vi "Address Claim.vi"(8 "error in (no error)":errorcluster, 11 "J1939 Main Configuration":T1={"Parameters"={"J1939 XNET Settings"={"XNET Database"="", "XNET Cluster"="", "CAN Port"="", "Baud rate [Bd]"=0, "Termination"=0, "Incoming Rate"=0, "Outcoming Rate"=1, "Write Decimation"=1}, "Incoming Single Point Configuraiton"={"Incoming Single Point Frame"={"ID"=[], "Conversion"=[], "Channel Array Positions"=[], "Frame Length"=[]}, "Channel Pairs"={"Chan Refs"=[], "Previous Chan Values"=[]}, "Read FIFO"=refnum}, "Outgoing Cyclic Configuraiton"={"Outgoing Cyclic Frame"={"ID"=[], "Conversion"=[], "Channel Array Positions"=[], "Frame Length"=[], "Transmit Propreties"=[]}, "Channel Pairs"={"Block Data Refs"=[], "Previous Chan Values"=[]}, "Write FIFO"=refnum}, "J1939 Monitor Settings"={"J1939 Network Address"=0, "Name"=0}, "Simulated Addresses"=[], "Simulated Addresses LUT"=variant, "Name"=""}, "Name"="", "J1939 Cluster"={"Processed Incoming"=refnum, "Current Device Address"=0, "Processed Outgoing"=refnum, "Process Outgoing"=refnum, "Name"=0}, "References"={"BAM Buffer"=refnum, "CM Buffer"=refnum, "CM Gen"=refnum, "BAM Gen"=refnum, "Address Claims"=refnum, "RQST"=refnum}, "Frame In"="", "Frame Out"="", "Incoming Timeout"=0, "Outgoing Timeout"=0, "Listener ID"=refnum, "Process"=refnum, "Data Ref"=refnum, "Scale Ref"=refnum, "Incoming Direct Access"={"Offset"=0, "Length"=0}, "Outgoing Direct Access"={"Offset"=0, "Length"=0}, "TCP Mngr Ref"=refnum, "Name and Address"="", "Simulated Addresses"=[], "Simulated Addresses LUT"=variant} {"Simulated Addresses"."Simulated Addresses"."J1939 XNET Settings"."Name" format="%.0x"; "Simulated Addresses"."Simulated Addresses"."DM1 Data"."Data Reference" format="%.0x"; "Simulated Addresses"."Simulated Addresses"."DM1 Enable?"."Data Reference" format="%.0x"; "Simulated Addresses"."Simulated Addresses"."DM2 Data"."Data Reference" format="%.0x"; "Simulated Addresses"."Simulated Addresses"."DM2 Enable?"."Data Reference" format="%.0x"; "Parameters"."Simulated Addresses"."Simulated Addresses"."J1939 XNET Settings"."Name" format="%.0x"; "Parameters"."J1939 Monitor Settings"."Name" format="%.0x"; "Parameters"."Outgoing Cyclic Configuraiton"."Channel Pairs"."Block Data Refs"."Data Reference" format="%.0x"; "Parameters"."Outgoing Cyclic Configuraiton"."Outgoing Cyclic Frame"."Transmit Propreties"."Transmit Time" format="%#_p"; "Parameters"."J1939 XNET Settings"."Termination" items=["Off", "On"]; "Parameters"."Incoming Single Point Configuraiton"."Channel Pairs"."Chan Refs" format="%.0x"}) -> (0 "error out":errorcluster, 3 "J1939 Main Configuration Out":T1={"Parameters"={"J1939 XNET Settings"={"XNET Database"="", "XNET Cluster"="", "CAN Port"="", "Baud rate [Bd]"=0, "Termination"=0, "Incoming Rate"=0, "Outcoming Rate"=1, "Write Decimation"=1}, "Incoming Single Point Configuraiton"={"Incoming Single Point Frame"={"ID"=[], "Conversion"=[], "Channel Array Positions"=[], "Frame Length"=[]}, "Channel Pairs"={"Chan Refs"=[], "Previous Chan Values"=[]}, "Read FIFO"=refnum}, "Outgoing Cyclic Configuraiton"={"Outgoing Cyclic Frame"={"ID"=[], "Conversion"=[], "Channel Array Positions"=[], "Frame Length"=[], "Transmit Propreties"=[]}, "Channel Pairs"={"Block Data Refs"=[], "Previous Chan Values"=[]}, "Write FIFO"=refnum}, "J1939 Monitor Settings"={"J1939 Network Address"=0, "Name"=0}, "Simulated Addresses"=[], "Simulated Addresses LUT"=variant, "Name"=""}, "Name"="", "J1939 Cluster"={"Processed Incoming"=refnum, "Current Device Address"=0, "Processed Outgoing"=refnum, "Process Outgoing"=refnum, "Name"=0}, "References"={"BAM Buffer"=refnum, "CM Buffer"=refnum, "CM Gen"=refnum, "BAM Gen"=refnum, "Address Claims"=refnum, "RQST"=refnum}, "Frame In"="", "Frame Out"="", "Incoming Timeout"=0, "Outgoing Timeout"=0, "Listener ID"=refnum, "Process"=refnum, "Data Ref"=refnum, "Scale Ref"=refnum, "Incoming Direct Access"={"Offset"=0, "Length"=0}, "Outgoing Direct Access"={"Offset"=0, "Length"=0}, "TCP Mngr Ref"=refnum, "Name and Address"="", "Simulated Addresses"=[], "Simulated Addresses LUT"=variant} {"Simulated Addresses"."Simulated Addresses"."J1939 XNET Settings"."Name" format="%.0x"; "Simulated Addresses"."Simulated Addresses"."DM1 Data"."Data Reference" format="%.0x"; "Simulated Addresses"."Simulated Addresses"."DM1 Enable?"."Data Reference" format="%.0x"; "Simulated Addresses"."Simulated Addresses"."DM2 Data"."Data Reference" format="%.0x"; "Simulated Addresses"."Simulated Addresses"."DM2 Enable?"."Data Reference" format="%.0x"; "Parameters"."Simulated Addresses"."Simulated Addresses"."J1939 XNET Settings"."Name" format="%.0x"; "Parameters"."J1939 Monitor Settings"."Name" format="%.0x"; "Parameters"."Outgoing Cyclic Configuraiton"."Channel Pairs"."Block Data Refs"."Data Reference" format="%.0x"; "Parameters"."Outgoing Cyclic Configuraiton"."Outgoing Cyclic Frame"."Transmit Propreties"."Transmit Time" format="%#_p"; "Parameters"."J1939 XNET Settings"."Termination" items=["Off", "On"]; "Parameters"."Incoming Single Point Configuraiton"."Channel Pairs"."Chan Refs" format="%.0x"})   [LabVIEW 2015, in "J1939 Addon Engine.lvlib"]
uses:
  J1939 Addon Engine.lvlib
  Types/Configuration Cluster.ctl
  <vilib>/NI/NI VeriStand Inline Async API/_VS Inline Async API/Process/Process.lvclass
  Types/Process Parameters.ctl
  Shared/Types/XNET Settings.ctl
  Types/Incoming Single Point Configuration.ctl
  Types/Incoming Single Point Frame Pairs.ctl
  Shared/Types/Incoming Single Point Channel Pairs.ctl
  <vilib>/NI Veristand/Custom Device API/Data Reference.ctl
  Types/Outgoing Cyclic Configuration.ctl
  Types/Outgoing Cyclic Frame Pairs.ctl
  Shared/Types/XNET Frame Event Properties.ctl
  Shared/Types/Outgoing Cyclic Channel Pairs.ctl
  <vilib>/NI Veristand/Custom Device API/Block Data Reference.ctl
  Shared/Types/Monitor Settings.ctl
  Types/Simulated Settings.ctl
  Shared/Types/Compiled Simulated Settings.ctl
  Types/DTC FIFOs.ctl
  Types/Setup Information Cluster.ctl
  <vilib>/xnet/xnet.llb/XNET Frame CAN.ctl
  <vilib>/xnet/xnet.llb/XNET Frame Type CAN.ctl
  Shared/J1939 Utilities/Types/CAN Outgoing Message Cluster.ctl
  Types/TP List References.ctl
  Types/BAM Buffer Connections List_Ref.ctl
  Types/TP Buffer Connection Cluster.ctl
  Types/Connection Mode Generation Connection Ref.ctl
  Types/Connection Mode Generation Connection Cluster.ctl
  Types/BAM Generation Connections List_Ref.ctl
  Types/BAM Generation Connection Cluster.ctl
  Types/Address Table Reference.ctl
  Types/RQST Lookup Table Reference.ctl
  Types/Data Lookup Table Reference.ctl
  Types/Datatable Lookup DVR.ctl
  Types/Conversion Lookup Table Reference.ctl
  Shared/Types/RQST Comm Lookup Table_Ref.ctl
  Shared/STM/Connection Manager/stm_ManagerStateVariables.ctl
  Shared/STM/TCP/stm_TCP Connection Info.ctl
  Shared/STM/_SubVIs/stm_MetaDataElement.ctl
  Shared/STM/Connection Manager/stm_TCPConnectionProperties.ctl
  Types/Address Lookup Table Action.ctl
  Shared/J1939 Utilities/SubVIs/Convert CAN Data (U8) to U32.vi
  Shared/J1939 Utilities/SubVIs/Convert CAN Data (U32) to U8.vi
  Shared/J1939 Utilities/SubVIs/Convert CAN Arb ID to J1939 ID.vi
  Shared/J1939 Utilities/SubVIs/Convert J1939 ID to CAN Arb ID.vi
  <vilib>/xnet/xnet.llb/XNET Write (Frame CAN).vi
  SubVIs/Address Lookup Table.vi
  <vilib>/xnet/xnet.llb/XNET Read.vi
  <vilib>/xnet/xnet.llb/XNET Read (Frame CAN).vi
  Shared/J1939 Utilities/SubVIs/Request Address.vi
  Shared/J1939 Utilities/J1939 Utilities.lvlib
  <vilib>/NI Veristand/Custom Device Tools/Custom Device Utility Library/Custom Device Utility Library.lvlib
  <vilib>/NI VeriStand/Custom Device API/Custom Device API.lvlib
  Shared/J1939 Addon Shared.lvlib
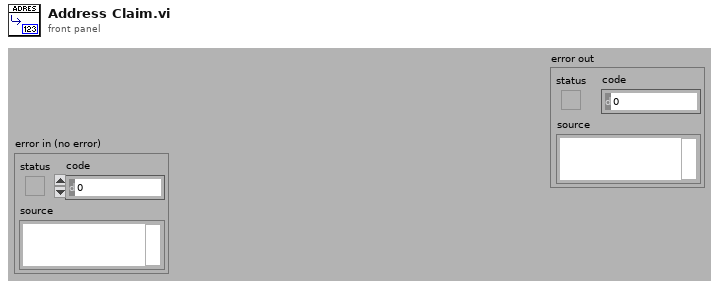
[diagram p1: front panel]
types:
  T1 = typedef "J1939 Addon Engine.lvlib/Configuration Cluster.ctl" = cluster{"Parameters":T2, "Name":string, "J1939 Cluster":T17, "References":T18, "Frame In":refnum<k21>, "Frame Out":refnum<k21>, "Incoming Timeout":u32, "Outgoing Timeout":u32, "Listener ID":refnum<k5>, "Process":refnum<class "Process.lvclass">, "Data Ref":T24, "Scale Ref":T25, "Incoming Direct Access":cluster{"Offset":u32, "Length":u32}, "Outgoing Direct Access":cluster{"Offset":u32, "Length":u32}, "TCP Mngr Ref":T26, "Name and Address":string, "Simulated Addresses":T14[], "Simulated Addresses LUT":variant}
  T2 = typedef "J1939 Addon Engine.lvlib/Process Parameters.ctl" = cluster{"J1939 XNET Settings":T3, "Incoming Single Point Configuraiton":T4, "Outgoing Cyclic Configuraiton":T8, "J1939 Monitor Settings":T13, "Simulated Addresses":T14[], "Simulated Addresses LUT":variant, "Name":string}
  T3 = typedef "J1939 Addon Shared.lvlib/XNET Settings.ctl" = cluster{"XNET Database":refnum<k21>, "XNET Cluster":refnum<k21>, "CAN Port":string, "Baud rate [Bd]":u32, "Termination":u32, "Incoming Rate":u32, "Outcoming Rate":u32, "Write Decimation":u32}
  T4 = typedef "J1939 Addon Engine.lvlib/Incoming Single Point Configuration.ctl" = cluster{"Incoming Single Point Frame":T5, "Channel Pairs":T6, "Read FIFO":refnum<k33>}
  T5 = typedef "J1939 Addon Engine.lvlib/Incoming Single Point Frame Pairs.ctl" = cluster{"ID":u32[], "Conversion":refnum<k21>[], "Channel Array Positions":cluster{"Offset":u32, "Length":u32}[], "Frame Length":u32[]}
  T6 = typedef "J1939 Addon Shared.lvlib/Incoming Single Point Channel Pairs.ctl" = cluster{"Chan Refs":T7[], "Previous Chan Values":dbl[]}
  T7 = typedef "Custom Device API.lvlib/Data Reference.ctl" = i32
  T8 = typedef "J1939 Addon Engine.lvlib/Outgoing Cyclic Configuration.ctl" = cluster{"Outgoing Cyclic Frame":T9, "Channel Pairs":T11, "Write FIFO":refnum<k33>}
  T9 = typedef "J1939 Addon Engine.lvlib/Outgoing Cyclic Frame Pairs.ctl" = cluster{"ID":u32[], "Conversion":refnum<k21>[], "Channel Array Positions":cluster{"Offset":u32, "Length":u32}[], "Frame Length":u32[], "Transmit Propreties":T10[]}
  T10 = typedef "J1939 Addon Shared.lvlib/XNET Frame Event Properties.ctl" = cluster{"Transmit trigger":enum16{"Channel value change"}, "Enable software cyclic trigger":bool, "Transmit Time":dbl}
  T11 = typedef "J1939 Addon Shared.lvlib/Outgoing Cyclic Channel Pairs.ctl" = cluster{"Block Data Refs":T12[], "Previous Chan Values":dbl[]}
  T12 = typedef "Custom Device API.lvlib/Block Data Reference.ctl" = cluster{"Data Reference":T7, "Offset":u64, "Length":u64}
  T13 = typedef "J1939 Addon Shared.lvlib/Monitor Settings.ctl" = cluster{"J1939 Network Address":u8, "Name":u64}
  T14 = typedef "J1939 Addon Engine.lvlib/Simulated Settings.ctl" = cluster{"Simulated Addresses":T15, "FIFOs":T16}
  T15 = typedef "J1939 Addon Shared.lvlib/Compiled Simulated Settings.ctl" = cluster{"J1939 XNET Settings":T13, "DM1 Data":T12[], "DM1 Data":dbl[], "DM1 Enable?":T12[], "DM1 Enable?":dbl[], "DM2 Data":T12[], "DM2 Data":dbl[], "DM2 Enable?":T12[], "DM2 Enable?":dbl[]}
  T16 = typedef "J1939 Addon Engine.lvlib/DTC FIFOs.ctl" = cluster{"DM1 Data":refnum<k33>, "DM1 Enable?":refnum<k33>, "DM2 Data":refnum<k33>, "DM2 Enable?":refnum<k33>, "DM1 Reset?":refnum<k33>, "DM2 Reset?":refnum<k33>}
  T17 = typedef "J1939 Addon Engine.lvlib/Setup Information Cluster.ctl" = cluster{"Processed Incoming":refnum<queue>, "Current Device Address":u8, "Processed Outgoing":refnum<queue>, "Process Outgoing":refnum<queue>, "Name":u64}
  T18 = typedef "J1939 Addon Engine.lvlib/TP List References.ctl" = cluster{"BAM Buffer":T19, "CM Buffer":T19, "CM Gen":T20, "BAM Gen":T21, "Address Claims":T22, "RQST":T23}
  T19 = typedef "J1939 Addon Engine.lvlib/BAM Buffer Connections List_Ref.ctl" = refnum<data-value>
  T20 = typedef "J1939 Addon Engine.lvlib/Connection Mode Generation Connection Ref.ctl" = refnum<data-value>
  T21 = typedef "J1939 Addon Engine.lvlib/BAM Generation Connections List_Ref.ctl" = refnum<data-value>
  T22 = typedef "J1939 Addon Engine.lvlib/Address Table Reference.ctl" = refnum<data-value>
  T23 = typedef "J1939 Addon Engine.lvlib/RQST Lookup Table Reference.ctl" = refnum<data-value>
  T24 = typedef "J1939 Addon Engine.lvlib/Data Lookup Table Reference.ctl" = refnum<data-value>
  T25 = typedef "J1939 Addon Engine.lvlib/Conversion Lookup Table Reference.ctl" = refnum<data-value>
  T26 = typedef "J1939 Addon Shared.lvlib/RQST Comm Lookup Table_Ref.ctl" = refnum<data-value>
  T27 = typedef "J1939 Addon Shared.lvlib/J1939 Utilities.lvlib/CAN Outgoing Message Cluster.ctl" = cluster{"Identifier":u32, "Data":u8[]}
  T28 = typedef "XNET Frame CAN.ctl" = cluster{"timestamp":timestamp, "payload":u8[], "identifier":u32, "type":T29, "extended?":bool, "echo?":bool}
  T29 = typedef "XNET Frame Type CAN.ctl" = u8
  T30 = typedef "J1939 Addon Shared.lvlib/J1939 Utilities.lvlib/Convert CAN Data (U8) Cluster.ctl" = cluster{"Byte 1":u8, "Byte 2":u8, "Byte 3":u8, "Byte 4":u8, "Byte 5":u8, "Byte 6":u8, "Byte 7":u8, "Byte 8":u8}
  T31 = typedef "J1939 Addon Engine.lvlib/Address Lookup Table Action.ctl" = enum16{"Initialize", "Add", "Get", "Remove", "Get All"}
  T32 = typedef "J1939 Addon Shared.lvlib/Address Lookup Table Data.ctl" = cluster{"Name":u8[], "Address":u8}
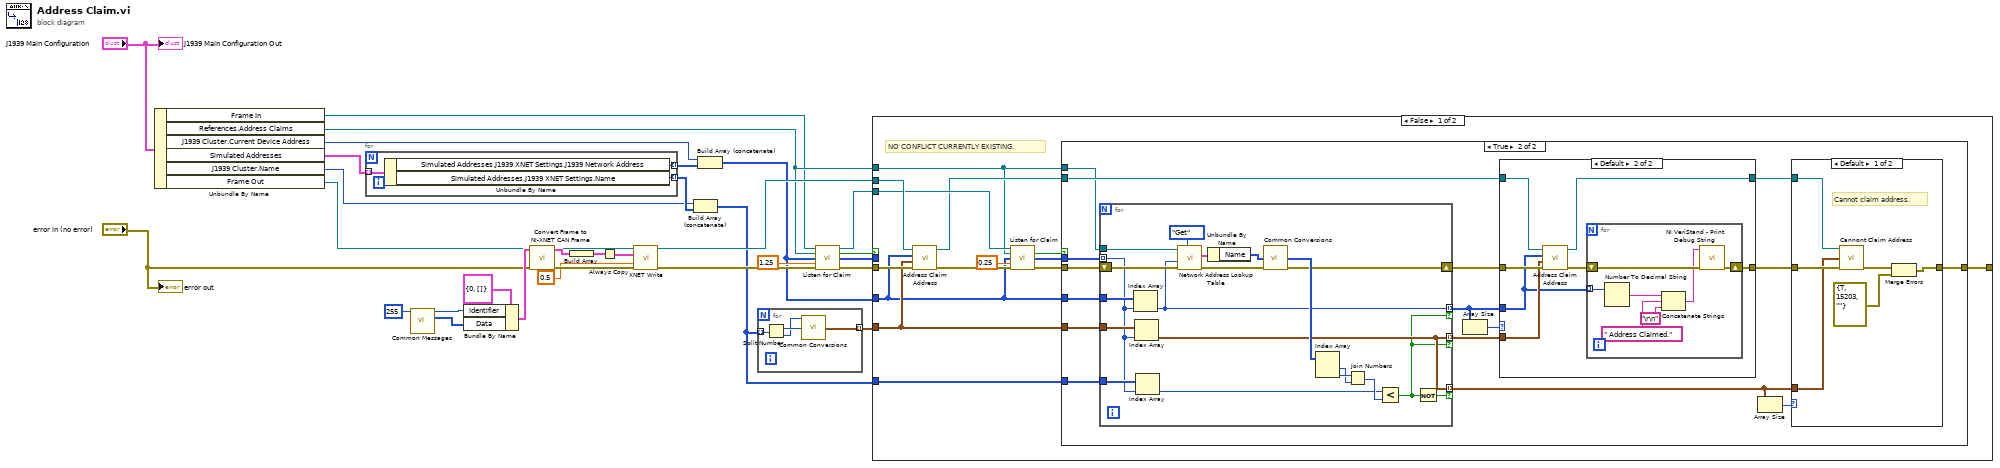
[diagram p0: block diagram]
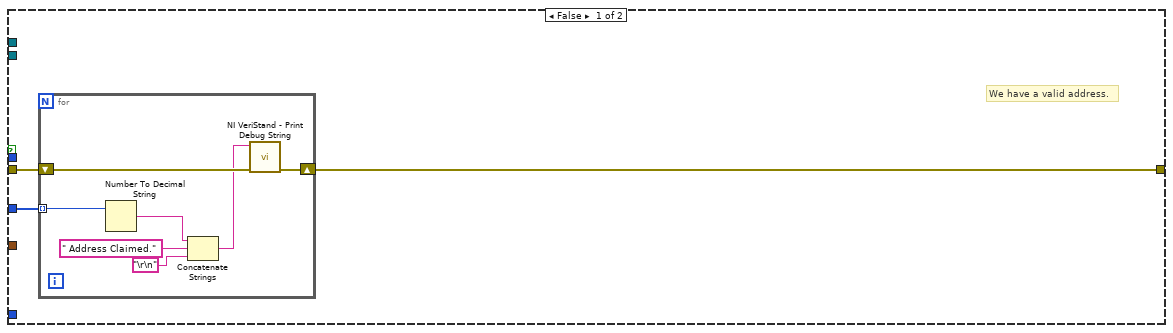
[diagram p2: hidden frame]
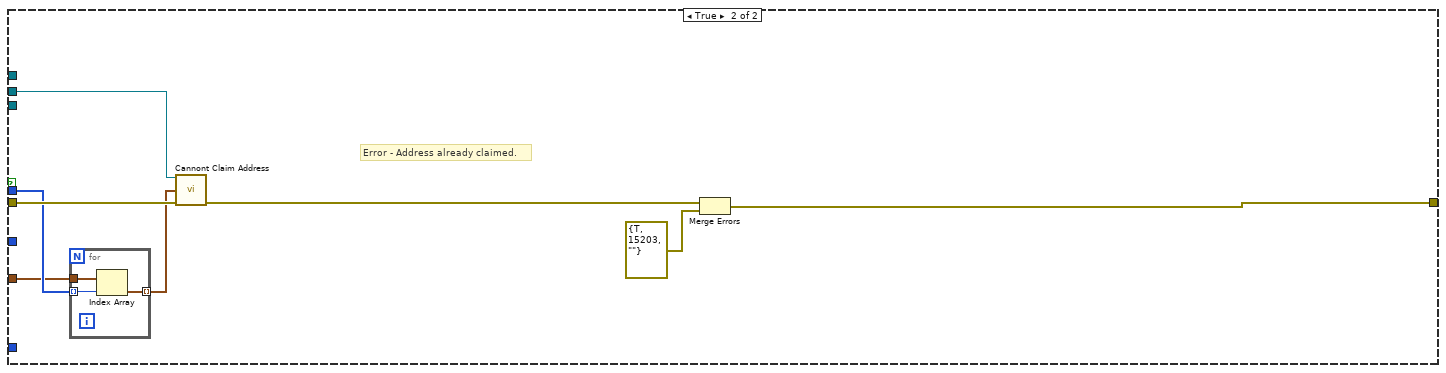
[diagram p5: hidden frame]
diagram:
  n1 = Unbundle By Name("J1939 Main Configuration") -> ("Frame In"=w1:refnum<k21>, "References.Address Claims"=w12:T22, "J1939 Cluster.Current Device Address"=w11:u8, "Simulated Addresses"=w7:T14[], "J1939 Cluster.Name"=w4:u64, "Frame Out"=w2:refnum<k21>)
  n2 = for {
    tunnel: w7 -> [w33] mode=indexing
    tunnel: [w31] -> w6 mode=indexing
    tunnel: [w32] -> w5 mode=indexing
    n3 = Unbundle By Name(w33) -> ("Simulated Addresses.J1939 XNET Settings.J1939 Network Address"=w31:u8, "Simulated Addresses.J1939 XNET Settings.Name"=w32:u64)
  }
  n4 = call-poly "Common Messages.vi"("Destination Address"=u8 255) -> ("Arb ID"=w30:u32, "Data"=w29:u8[])  [unwired: 13 in]
  n5 = Bundle By Name(cluster=T27 {"Identifier"=0, "Data"=[]} ("Data to Send"), "Identifier"=w30, "Data"=w29) -> (w27:T27)
  n6 = call "Convert Frame to NI-XNET CAN Frame.vi"("error in (no error)"="error in (no error)", "Data to Send"=w27) -> ("error out"=w25:errorcluster, "CAN frame"=w26:T28)  [unwired: 8 in]
  n7 = Build Array(w26) -> (w15:T28[])
  n8 = Always Copy(1:w15) -> (0:w10:T28[])
  n9 = call-poly <vilib>:"XNET Write.vi"("session in"=w2, "data"=w10, "timeout (10)"=0.5, "error in (no error)"=w25) -> ("session out"=w19:refnum<k21>, "error out"=w24:errorcluster)  [unwired: 10 out]
  n10 = Build Array (concatenate)(w4, w5) -> (w9:u64[])
  n11 = Build Array (concatenate)(w11, w6) -> (w3:u8[])
  n12 = for {
    tunnel: [w34] -> w18 mode=indexing
    tunnel: w9 -> [w35] mode=indexing
    n13 = Split Number(x=w35) -> (hi(x)=w37:u32, lo(x)=w36:u32)
    n14 = call-poly "Common Conversions.vi"("Data 0-3"=w36, "Data 4-7"=w37) -> ("Byte Cluster"=w34:T30)  [unwired: 13 in]
  }
  n15 = call "Listen for Claim.vi"("session in"=w1, "ref in"=w12, "Requested Addresses"=w3, "timeout (0)"=1.25, "error in"=w24) -> ("session out"=w21:refnum<k21>, "Conflict?"=w22:bool, "Conflict Indeces"=w8:i32[], "error out"=w20:errorcluster)  [unwired: 7 in]
  n16 = case shown="False" w22 {
    tunnel: w3 -> [w39 _]
    tunnel: w9 -> [w46 _]
    tunnel: w21 -> [w48 _]
    tunnel: w20 -> [w49 w127]
    tunnel: w19 -> [w50 w126]
    tunnel: [w42 w123] -> _
    tunnel: w18 -> [w41 w121]
    tunnel: w12 -> [w40 _]
    tunnel: w8 -> [_ w122]
    frame False {
      # "NO CONFLICT CURRENTLY EXISTING."
      n17 = call "Address Claim Address.vi"("error in"=w49, "Names"=w41, "Requested Addresses"=w39, "session in"=w50) -> ("error out"=w51:errorcluster, "session out"=w44:refnum<k21>)  [unwired: 6 in]
      n18 = call "Listen for Claim.vi"("session in"=w48, "ref in"=w40, "Requested Addresses"=w39, "timeout (0)"=0.25, "error in"=w51) -> ("Conflict?"=w45:bool, "Conflict Indeces"=w38:i32[], "error out"=w43:errorcluster)  [unwired: 7 in, 1 out]
      n19 = case shown="True" w45 {
        tunnel: w46 -> [_ w69]
        tunnel: w44 -> [_ w77]
        tunnel: w43 -> [w54 w76]
        tunnel: w41 -> [_ w71]
        tunnel: [w53 w64] -> w42
        tunnel: w40 -> [_ w74]
        tunnel: w39 -> [w52 w70]
        tunnel: w38 -> [_ w73]
        frame False {
          # "We have a valid address."
          n20 = for {
            shift-right: [w60] -> w53
            shift-left: w54 -> [w61]
            tunnel: w52 -> [w57] mode=indexing
            n21 = Number To Decimal String(number=w57) -> (decimal integer string=w56:string)  [unwired: 1 in]
            n22 = Concatenate Strings(w56, " Address Claimed." ("string"), "\r\n") -> (w58:string)
            n23 = call <vilib>:"NI VeriStand - Print Debug String.vi"("error in (no error)"=w61, "Message"=w58) -> ("error out"=w60:errorcluster)  [unwired: 9 in]
          }
        }
        frame True {
          n24 = for {
            tunnel: w74 -> [w96]
            tunnel: w73 -> [w87] mode=indexing
            tunnel: [w89] -> w72 mode=indexing if=w86
            tunnel: w71 -> [w93]
            tunnel: w70 -> [w92]
            tunnel: [w85] -> w68 mode=indexing if=w86
            tunnel: w69 -> [w91]
            shift-right: [w97] -> w75
            shift-left: w76 -> [w98]
            tunnel: [w89] -> w62 mode=indexing if=w88
            n25 = Index Array(array=w92, index=w87) -> (element=w85:u8)
            n26 = Index Array(array=w93, index=w87) -> (element=w89:T30)
            n27 = Index Array(array=w91, index=w87) -> (element=w90:u64)
            n28 = call "Network Address Lookup Table.vi"("Action"=Address_Lookup_Table_Action."Get", "error in (no error)"=w98, "Address"=w85, "Address LUT"=w96) -> ("error out"=w97:errorcluster, "Data"=w95:T32)  [unwired: 3 in, 3 out]
            n29 = Unbundle By Name(w95) -> ("Name"=w94:u8[])
            n30 = call-poly "Common Conversions.vi"("Data"=w94) -> ("Array"=w103:u32[])  [unwired: 14 in]
            n31 = Index Array(array=w103) -> (element #1=w101:u32, element #2=w102:u32)  [unwired: 2 in]
            n32 = Join Numbers(hi=w102, lo=w101) -> ((hi.lo)=w100:u64)
            n33 = Less?(x=w90, y=w100) -> (x < y?=w86:bool)
            n34 = Not(x=w86) -> (.not. x?=w88:bool)
          }
          n35 = Array Size(array=w68) -> (size(s)=w67:i32)
          n36 = case shown="Default" w67 {
            tunnel: w77 -> [w104 w111]
            tunnel: w75 -> [w105 w112]
            tunnel: w72 -> [_ w110]
            tunnel: [w105 w108] -> w65
            tunnel: w68 -> [_ w106]
            tunnel: [w104 w107] -> w66
            frame 0 {
            }
            frame Default {
              n37 = call "Address Claim Address.vi"("error in"=w112, "Names"=w110, "Requested Addresses"=w106, "session in"=w111) -> ("error out"=w109:errorcluster, "session out"=w107:refnum<k21>)  [unwired: 6 in]
              n38 = for {
                shift-right: [w118] -> w108
                shift-left: w109 -> [w119]
                tunnel: w106 -> [w117] mode=indexing
                n39 = Number To Decimal String(number=w117) -> (decimal integer string=w116:string)  [unwired: 1 in]
                n40 = Concatenate Strings(w116, " Address Claimed." ("string"), "\r\n") -> (w115:string)
                n41 = call <vilib>:"NI VeriStand - Print Debug String.vi"("error in (no error)"=w119, "Message"=w115) -> ("error out"=w118:errorcluster)  [unwired: 9 in]
              }
            }
          }
          n42 = Array Size(array=w62) -> (size(s)=w63:i32)
          n43 = case shown="Default" w63 {
            tunnel: w66 -> [w81 _]
            tunnel: w65 -> [w83 w84]
            tunnel: w62 -> [w82 _]
            tunnel: [w78 w84] -> w64
            frame Default {
              # "Cannot claim address."
              n44 = call "Cannont Claim Address.vi"("session out"=w81, "Names"=w82, "error in"=w83) -> ("error out"=w80:errorcluster)  [unwired: 12 in]
              n45 = Merge Errors(w80, errorcluster {"status"=TRUE, "code"=15203, "source"=""} ("error out")) -> (w78:errorcluster)
            }
            frame 0 {
            }
          }
        }
      }
    }
    frame True {
      # "Error - Address already claimed."
      n46 = for {
        tunnel: w122 -> [w129] mode=indexing
        tunnel: w121 -> [w130]
        tunnel: [w128] -> w120 mode=indexing
        n47 = Index Array(array=w130, index=w129) -> (element=w128:T30)
      }
      n48 = call "Cannont Claim Address.vi"("session out"=w126, "Names"=w120, "error in"=w127) -> ("error out"=w124:errorcluster)  [unwired: 12 in]
      n49 = Merge Errors(w124, errorcluster {"status"=TRUE, "code"=15203, "source"=""} ("error out")) -> (w123:errorcluster)
    }
  }
  "error out" <- "error in (no error)"
  "J1939 Main Configuration Out" <- "J1939 Main Configuration"
